vi "Logger Not Initialized Error Constant.vi"() -> (0 "Logger Not Initialized Error":errorcluster)   [LabVIEW 2020, in "hse-logger.lvlib"]
doc: "____\nHAMPEL SOFTWARE ENGINEERING v2.0.6 (2021-04-15 11:38)"
uses:
  hse-logger.lvlib
  <vilib>/ErrorRing/Error Ring.xnode
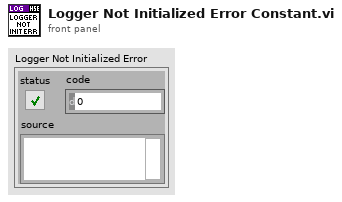
[diagram p1: front panel]
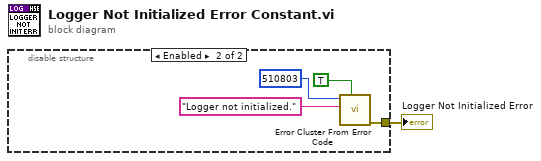
[diagram p0: block diagram]
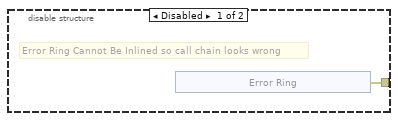
[diagram p2: hidden frame]
diagram:
  n1 = disable-structure shown="Enabled" {
    disable-tunnel: [w2 w8] -> w1
    frame Disabled {
      # "Error Ring Cannot Be Inlined so call chain looks wrong"
      n2 = xnode "Error Ring"() -> ("error out"=w2:errorcluster)
    }
    frame Enabled {
      n3 = call <vilib>:"Error Cluster From Error Code.vi"("show call chain? (False)"=TRUE, "error message (\"\")"="Logger not initialized." ("error message (\"\")"), "error code (0)"=510803) -> ("error out"=w8:errorcluster)  [unwired: 6 in]
    }
  }
  "Logger Not Initialized Error" <- w1
